vi "Actor Core.vi"(8 "error in":errorcluster, 11 "XBoxController-P in":refnum<class "XBoxController-P.lvclass">) -> (0 "error out":errorcluster, 3 "Actor out":refnum<class "Actor.lvclass">)   [LabVIEW 2013, in "XBoxController-P.lvclass"]
doc: "(<B>Filename</B>: Actor Framework.lvlib:Actor.lvclass:Actor Core.vi)\n\nReceives messages to the actor, reacts to them, and initiates any error handling that may shut the actor down.\n\nDescendant classes may override this VI to append parallel tasks for the actor to complete while it handles messages. Overrides use the Call Parent Method node."
uses:
  XBoxController-P.lvclass
  <vilib>/ActorFramework/Actor/Actor.lvclass
  <vilib>/Rock Robotics/WPI/Joystick/WPI_JoystickButtonState.ctl
  XBoxController-P.lvclass/XBoxController-P.ctl
  Logical Systems/XBoxController/XBoxController.lvclass
panel:
  out "Buttons":T1
  out "Axes":T2
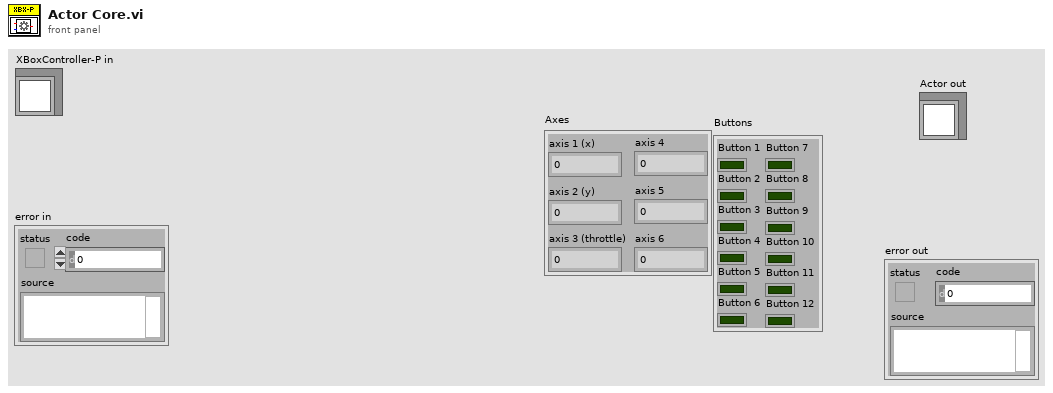
[diagram p1: front panel]
types:
  T1 = typedef "WPI_JoystickButtonState.ctl" = cluster{"Button 1":bool, "Button 2":bool, "Button 3":bool, "Button 4":bool, "Button 5":bool, "Button 6":bool, "Button 7":bool, "Button 8":bool, "Button 9":bool, "Button 10":bool, "Button 11":bool, "Button 12":bool}
  T2 = cluster{"axis 1 (x)":dbl, "axis 2 (y)":dbl, "axis 3 (throttle)":dbl, "axis 4":dbl, "axis 5":dbl, "axis 6":dbl}
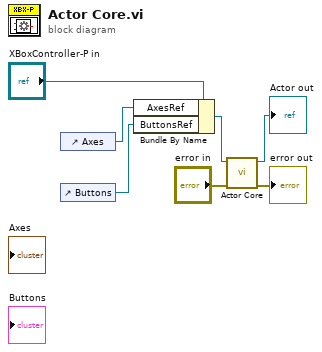
[diagram p0: block diagram]
diagram:
  n1 = control-ref of="Axes"() -> (w2:refnum<vi>)
  n2 = control-ref of="Buttons"() -> (w1:refnum<vi>)
  n3 = Bundle By Name(cluster="XBoxController-P in", "AxesRef"=w2, "ButtonsRef"=w1) -> (w3:refnum<class "XBoxController-P.lvclass">)
  n4 = call-parent "Actor Core.vi"("error in"="error in", "XBoxController in"=w3) -> ("error out"=→"error out":errorcluster, "Actor out"=→"Actor out":refnum<class "Actor.lvclass">)  [unwired: 8 in]
